vi "Lab Panel V4.82.vi"() -> ()   [LabVIEW 2013] (continued)
                        n2459 = call "sub vi - send mail with attach v5.vi"("TO:"=w4136, "subject"="MAIL TEST FROM LAB PANEL", "from"=w4135, "out going server"=w4134, "message"="TEST MESSAGE") -> ("error out"=w4138:errorcluster)  [unwired: 10 in]
                      }
                      frame #3 {
                        n2460 = Bundle(cluster=w4143, "TEST MAIL"=FALSE, "TEST MAIL STATUS"="TEST END", "mail error"=w4139) -> (w4141:T7)  [unwired: 4 in]
                        n2461 = local write "MAIL SETTINGS"(w4141) -> ()
                      }
                    }
                  }
                }
              }
              frame #1 {
                # "mail report"
                n2462 = stacked-sequence {
                  seq-local: [_ w4223 _ _] -> [_ _ _ w4391]
                  seq-local: [_ _ w4304 _] -> [_ _ _ w4381]
                  seq-local: [w4168 _ _ _] -> [_ w4217 _ _]
                  seq-local: [w4167 _ _ _] -> [_ w4216 _ _]
                  seq-local: [w4165 _ _ _] -> [_ w4214 _ _]
                  seq-local: [w4166 _ _ _] -> [_ w4215 _ _]
                  seq-local: [w4164 _ _ _] -> [_ w4213 _ _]
                  seq-local: [w4163 _ _ _] -> [_ w4208 _ _]
                  seq-local: [w4162 _ _ _] -> [_ w4209 _ _]
                  seq-local: [w4161 _ _ _] -> [_ w4210 _ _]
                  seq-local: [w4160 _ _ _] -> [_ w4211 _ _]
                  seq-local: [w4159 _ _ _] -> [_ w4212 _ _]
                  tunnel: w4158 -> [_ _ _ w4392]
                  tunnel: w4157 -> [_ _ _ w4375]
                  tunnel: w4156 -> [_ _ _ w4389]
                  tunnel: w4155 -> [_ _ _ w4388]
                  tunnel: w4154 -> [w4199 _ _ w4383]
                  tunnel: w4153 -> [_ _ w4334 _]
                  tunnel: w4152 -> [_ _ w4331 _]
                  tunnel: w4151 -> [_ _ w4330 _]
                  tunnel: w4150 -> [_ _ w4329 _]
                  tunnel: w4149 -> [_ _ w4328 _]
                  tunnel: w4148 -> [_ _ w4327 _]
                  tunnel: w4147 -> [_ _ w4326 _]
                  tunnel: w4146 -> [_ _ w4325 _]
                  tunnel: w4145 -> [_ _ w4324 _]
                  tunnel: w4144 -> [_ _ w4323 _]
                  frame #0 {
                    n2463 = case shown="False" w4199 {
                      frame False {
                        n2464 = local write "mail control"("") -> ()
                      }
                      frame True {
                      }
                    }
                    n2465 = local read "SET LAB01-1"() -> (w4198:T5)
                    n2466 = local read "SET LAB01-2"() -> (w4197:T5)
                    n2467 = local read "SET LAB02-1"() -> (w4196:T5)
                    n2468 = local read "SET LAB02-2"() -> (w4195:T5)
                    n2469 = local read "SET LAB03-1"() -> (w4194:T5)
                    n2470 = local read "SET LAB04-1"() -> (w4192:T5)
                    n2471 = local read "SET LAB05-1"() -> (w4190:T5)
                    n2472 = local read "SET LAB03-2"() -> (w4193:T5)
                    n2473 = local read "SET LAB04-2"() -> (w4191:T5)
                    n2474 = local read "SET LAB05-2"() -> (w4189:T5)
                    n2475 = Unbundle(w4194) -> ("DESCRIPTION"=w4174:string)  [unwired: 4 out]
                    n2476 = Unbundle(w4193) -> ("DESCRIPTION"=w4173:string)  [unwired: 4 out]
                    n2477 = Unbundle(w4192) -> ("DESCRIPTION"=w4172:string)  [unwired: 4 out]
                    n2478 = Unbundle(w4189) -> ("DESCRIPTION"=w4169:string)  [unwired: 4 out]
                    n2479 = Unbundle(w4195) -> ("DESCRIPTION"=w4175:string)  [unwired: 4 out]
                    n2480 = Unbundle(w4191) -> ("DESCRIPTION"=w4171:string)  [unwired: 4 out]
                    n2481 = Unbundle(w4198) -> ("DESCRIPTION"=w4187:string)  [unwired: 4 out]
                    n2482 = Unbundle(w4196) -> ("DESCRIPTION"=w4176:string)  [unwired: 4 out]
                    n2483 = Unbundle(w4190) -> ("DESCRIPTION"=w4170:string)  [unwired: 4 out]
                    n2484 = Unbundle(w4197) -> ("DESCRIPTION"=w4177:string)  [unwired: 4 out]
                    n2485 = Concatenate Strings("[LAB05-2/", w4169) -> (w4159:string)
                    n2486 = Concatenate Strings("[LAB05-1/", w4170) -> (w4160:string)
                    n2487 = Concatenate Strings("[LAB04-2/", w4171) -> (w4161:string)
                    n2488 = Concatenate Strings("[LAB03-2/", w4173) -> (w4163:string)
                    n2489 = Concatenate Strings("[LAB04-1/", w4172) -> (w4162:string)
                    n2490 = Concatenate Strings("[LAB03-1/", w4174) -> (w4164:string)
                    n2491 = Concatenate Strings("[LAB01-2/", w4177) -> (w4167:string)
                    n2492 = Concatenate Strings("[LAB02-2/", w4175) -> (w4165:string)
                    n2493 = Concatenate Strings("[LAB01-1/", w4187) -> (w4168:string)
                    n2494 = Concatenate Strings("[LAB02-1/", w4176) -> (w4166:string)
                  }
                  frame #1 {
                    w4221 = "/"
                    w4222 = 2.0
                    n2495 = local read "DISP LAB01-2"() -> (w4302:T4)
                    n2496 = local read "DISP LAB01-1"() -> (w4303:T4)
                    n2497 = local read "DISP LAB02-1"() -> (w4301:T4)
                    n2498 = local read "DISP LAB03-2"() -> (w4298:T4)
                    n2499 = local read "DISP LAB02-2"() -> (w4300:T4)
                    n2500 = local read "DISP LAB03-1"() -> (w4299:T4)
                    n2501 = local read "DISP LAB04-2"() -> (w4296:T4)
                    n2502 = local read "DISP LAB04-1"() -> (w4297:T4)
                    n2503 = local read "DISP LAB05-1"() -> (w4295:T4)
                    n2504 = local read "DISP LAB05-2"() -> (w4294:T4)
                    n2505 = Unbundle(w4302) -> ("CYCLE"=w4286:dbl, "MINS"=w4285:dbl, "STATUS"=w4282:string)
                    n2506 = Unbundle(w4303) -> ("CYCLE"=w4291:dbl, "MINS"=w4290:dbl, "STATUS"=w4287:string)
                    n2507 = Unbundle(w4301) -> ("CYCLE"=w4279:dbl, "MINS"=w4278:dbl, "STATUS"=w4277:string)
                    n2508 = Unbundle(w4298) -> ("CYCLE"=w4266:dbl, "MINS"=w4265:dbl, "STATUS"=w4262:string)
                    n2509 = Unbundle(w4299) -> ("CYCLE"=w4271:dbl, "MINS"=w4270:dbl, "STATUS"=w4267:string)
                    n2510 = Unbundle(w4300) -> ("CYCLE"=w4276:dbl, "MINS"=w4275:dbl, "STATUS"=w4272:string)
                    n2511 = Unbundle(w4297) -> ("CYCLE"=w4261:dbl, "MINS"=w4260:dbl, "STATUS"=w4257:string)
                    n2512 = Unbundle(w4296) -> ("CYCLE"=w4256:dbl, "MINS"=w4255:dbl, "STATUS"=w4252:string)
                    n2513 = Unbundle(w4295) -> ("CYCLE"=w4251:dbl, "MINS"=w4250:dbl, "STATUS"=w4247:string)
                    n2514 = Unbundle(w4294) -> ("CYCLE"=w4293:dbl, "MINS"=w4292:dbl, "STATUS"=w4244:string)
                    n2515 = Number To Decimal String(number=w4279) -> (decimal integer string=w4281:string)  [unwired: 1 in]
                    n2516 = Number To Decimal String(number=w4276) -> (decimal integer string=w4274:string)  [unwired: 1 in]
                    n2517 = Number To Decimal String(number=w4271) -> (decimal integer string=w4269:string)  [unwired: 1 in]
                    n2518 = Number To Decimal String(number=w4286) -> (decimal integer string=w4284:string)  [unwired: 1 in]
                    n2519 = Number To Decimal String(number=w4266) -> (decimal integer string=w4264:string)  [unwired: 1 in]
                    n2520 = Number To Decimal String(number=w4291) -> (decimal integer string=w4289:string)  [unwired: 1 in]
                    n2521 = Number To Decimal String(number=w4293) -> (decimal integer string=w4246:string)  [unwired: 1 in]
                    n2522 = Number To Decimal String(number=w4261) -> (decimal integer string=w4259:string)  [unwired: 1 in]
                    n2523 = Number To Decimal String(number=w4256) -> (decimal integer string=w4254:string)  [unwired: 1 in]
                    n2524 = Number To Decimal String(number=w4251) -> (decimal integer string=w4249:string)  [unwired: 1 in]
                    n2525 = Number To Fractional String(number=w4278, precision (6)=w4222) -> (F-format string=w4280:string)  [unwired: 2 in]
                    n2526 = Number To Fractional String(number=w4265, precision (6)=w4222) -> (F-format string=w4263:string)  [unwired: 2 in]
                    n2527 = Number To Fractional String(number=w4275, precision (6)=w4222) -> (F-format string=w4273:string)  [unwired: 2 in]
                    n2528 = Number To Fractional String(number=w4270, precision (6)=w4222) -> (F-format string=w4268:string)  [unwired: 2 in]
                    n2529 = Number To Fractional String(number=w4255, precision (6)=w4222) -> (F-format string=w4253:string)  [unwired: 2 in]
                    n2530 = Number To Fractional String(number=w4260, precision (6)=w4222) -> (F-format string=w4258:string)  [unwired: 2 in]
                    n2531 = Number To Fractional String(number=w4285, precision (6)=w4222) -> (F-format string=w4283:string)  [unwired: 2 in]
                    n2532 = Number To Fractional String(number=w4250, precision (6)=w4222) -> (F-format string=w4248:string)  [unwired: 2 in]
                    n2533 = Number To Fractional String(number=w4290, precision (6)=w4222) -> (F-format string=w4288:string)  [unwired: 2 in]
                    n2534 = Number To Fractional String(number=w4292, precision (6)=w4222) -> (F-format string=w4245:string)  [unwired: 2 in]
                    n2535 = Concatenate Strings(w4221, w4264, w4221, w4263, w4221, w4262) -> (w4238:string)
                    n2536 = Concatenate Strings(w4221, w4259, w4221, w4258, w4221, w4257) -> (w4237:string)
                    n2537 = Concatenate Strings(w4221, w4254, w4221, w4253, w4221, w4252) -> (w4236:string)
                    n2538 = Concatenate Strings(w4221, w4249, w4221, w4248, w4221, w4247) -> (w4235:string)
                    n2539 = Concatenate Strings(w4221, w4246, w4221, w4245, w4221, w4244) -> (w4234:string)
                    n2540 = Concatenate Strings(w4221, w4289, w4221, w4288, w4221, w4287) -> (w4243:string)
                    n2541 = Concatenate Strings(w4221, w4269, w4221, w4268, w4221, w4267) -> (w4239:string)
                    n2542 = Concatenate Strings(w4221, w4284, w4221, w4283, w4221, w4282) -> (w4242:string)
                    n2543 = Concatenate Strings(w4221, w4281, w4221, w4280, w4221, w4277) -> (w4241:string)
                    n2544 = Concatenate Strings(w4221, w4274, w4221, w4273, w4221, w4272) -> (w4240:string)
                    n2545 = Concatenate Strings("]", "\r") -> (w4218:string)
                    n2546 = Concatenate Strings(w4213, w4239, w4218) -> (w4229:string)
                    n2547 = Concatenate Strings(w4215, w4241, w4218) -> (w4231:string)
                    n2548 = Concatenate Strings(w4214, w4240, w4218) -> (w4230:string)
                    n2549 = Concatenate Strings(w4210, w4236, w4218) -> (w4226:string)
                    n2550 = Concatenate Strings(w4211, w4235, w4218) -> (w4227:string)
                    n2551 = Concatenate Strings(w4209, w4237, w4218) -> (w4225:string)
                    n2552 = Concatenate Strings(w4208, w4238, w4218) -> (w4224:string)
                    n2553 = Concatenate Strings(w4212, w4234, w4218) -> (w4228:string)
                    n2554 = Concatenate Strings(w4216, w4242, w4218) -> (w4232:string)
                    n2555 = Concatenate Strings(w4217, w4243, w4218) -> (w4233:string)
                    n2556 = Concatenate Strings(w4233, w4232, w4231, w4230, w4229, w4224, w4225, w4226, w4227, w4228) -> (w4201:string)
                    n2557 = Concatenate Strings("[PANEL/", "DESC/", "CYCLES/", "MINS/", "STATUS]", "\r", w4201) -> (w4223:string)
                    "MAIL REPORT" <- w4223
                  }
                  frame #2 {
                    w4332 = "END"
                    n2558 = local read "mail control"() -> (w4333:string)
                    n2559 = case shown="False" w4328 {
                      tunnel: w4333 -> [w4357 _]
                      tunnel: w4332 -> [w4356 _]
                      tunnel: [w4355 FALSE] -> w4318
                      frame False {
                        n2560 = Equal?(x=w4357, y=w4356) -> (x = y?=w4355:bool)
                      }
                      frame True {
                      }
                    }
                    n2561 = case shown="False" w4334 {
                      tunnel: w4333 -> [w4373 _]
                      tunnel: w4332 -> [w4372 _]
                      tunnel: [w4371 FALSE] -> w4322
                      frame False {
                        n2562 = Equal?(x=w4373, y=w4372) -> (x = y?=w4371:bool)
                      }
                      frame True {
                      }
                    }
                    n2563 = case shown="False" w4331 {
                      tunnel: w4333 -> [w4369 _]
                      tunnel: w4332 -> [w4368 _]
                      tunnel: [w4367 FALSE] -> w4321
                      frame False {
                        n2564 = Equal?(x=w4369, y=w4368) -> (x = y?=w4367:bool)
                      }
                      frame True {
                      }
                    }
                    n2565 = case shown="False" w4329 {
                      tunnel: w4333 -> [w4361 _]
                      tunnel: w4332 -> [w4360 _]
                      tunnel: [w4359 FALSE] -> w4319
                      frame False {
                        n2566 = Equal?(x=w4361, y=w4360) -> (x = y?=w4359:bool)
                      }
                      frame True {
                      }
                    }
                    n2567 = case shown="False" w4330 {
                      tunnel: w4333 -> [w4365 _]
                      tunnel: w4332 -> [w4364 _]
                      tunnel: [w4363 FALSE] -> w4320
                      frame False {
                        n2568 = Equal?(x=w4365, y=w4364) -> (x = y?=w4363:bool)
                      }
                      frame True {
                      }
                    }
                    n2569 = Or(x=w4320, y=w4319) -> (x .or. y?=w4311:bool)
                    n2570 = Or(x=w4322, y=w4321) -> (x .or. y?=w4312:bool)
                    n2571 = Or(x=w4312, y=w4311) -> (x .or. y?=w4307:bool)
                    n2572 = case shown="False" w4324 {
                      tunnel: w4333 -> [w4341 _]
                      tunnel: w4332 -> [w4340 _]
                      tunnel: [w4339 FALSE] -> w4313
                      frame False {
                        n2573 = Equal?(x=w4341, y=w4340) -> (x = y?=w4339:bool)
                      }
                      frame True {
                      }
                    }
                    n2574 = case shown="False" w4323 {
                      tunnel: w4333 -> [w4337 _]
                      tunnel: w4332 -> [w4336 _]
                      tunnel: [w4335 FALSE] -> w4317
                      frame False {
                        n2575 = Equal?(x=w4337, y=w4336) -> (x = y?=w4335:bool)
                      }
                      frame True {
                      }
                    }
                    n2576 = case shown="False" w4325 {
                      tunnel: w4333 -> [w4345 _]
                      tunnel: w4332 -> [w4344 _]
                      tunnel: [w4343 FALSE] -> w4314
                      frame False {
                        n2577 = Equal?(x=w4345, y=w4344) -> (x = y?=w4343:bool)
                      }
                      frame True {
                      }
                    }
                    n2578 = case shown="False" w4327 {
                      tunnel: w4333 -> [w4353 _]
                      tunnel: w4332 -> [w4352 _]
                      tunnel: [w4351 FALSE] -> w4316
                      frame False {
                        n2579 = Equal?(x=w4353, y=w4352) -> (x = y?=w4351:bool)
                      }
                      frame True {
                      }
                    }
                    n2580 = case shown="False" w4326 {
                      tunnel: w4333 -> [w4349 _]
                      tunnel: w4332 -> [w4348 _]
                      tunnel: [w4347 FALSE] -> w4315
                      frame False {
                        n2581 = Equal?(x=w4349, y=w4348) -> (x = y?=w4347:bool)
                      }
                      frame True {
                      }
                    }
                    n2582 = Or(x=w4316, y=w4315) -> (x .or. y?=w4310:bool)
                    n2583 = Or(x=w4314, y=w4313) -> (x .or. y?=w4309:bool)
                    n2584 = Or(x=w4317, y=w4318) -> (x .or. y?=w4305:bool)
                    n2585 = Or(x=w4310, y=w4309) -> (x .or. y?=w4308:bool)
                    n2586 = Or(x=w4307, y=w4308) -> (x .or. y?=w4306:bool)
                    n2587 = Or(x=w4306, y=w4305) -> (x .or. y?=w4304:bool)
                  }
                  frame #3 {
                    n2588 = local read "on loops"() -> (w4387:dbl)
                    n2589 = local read "jig cycle"() -> (w4384:dbl)
                    n2590 = local read "Send Mail Now"() -> (w4378:bool)
                    n2591 = Add(x=w4387, y=3.0) -> (x+y=w4385:dbl)
                    n2592 = Equal?(x=w4384, y=w4385) -> (x = y?=w4379:bool)
                    n2593 = And(x=w4379, y=w4378) -> (x .and. y?=w4377:bool)
                    n2594 = And(x=w4383, y=w4379) -> (x .and. y?=w4382:bool)
                    n2595 = And(x=w4382, y=w4381) -> (x .and. y?=w4380:bool)
                    n2596 = Or(x=w4380, y=w4377) -> (x .or. y?=w4376:bool)
                    n2597 = case shown="True" w4376 {
                      tunnel: w4392 -> [_ w4398]
                      tunnel: w4391 -> [_ w4397]
                      tunnel: "Lab Panel Test Status" -> [_ w4396]
                      tunnel: w4389 -> [_ w4395]
                      tunnel: w4388 -> [_ w4394]
                      tunnel: w4375 -> [_ w4393]
                      frame False {
                      }
                      frame True {
                        n2598 = stacked-sequence {
                          tunnel: w4398 -> [w4406 _]
                          tunnel: w4397 -> [w4405 _]
                          tunnel: w4396 -> [w4404 _]
                          tunnel: w4395 -> [w4403 _]
                          tunnel: w4394 -> [w4402 _]
                          tunnel: w4393 -> [w4401 _]
                          frame #0 {
                            n2599 = call "sub vi - send mail with attach v5.vi"("TO:"=w4406, "subject"=w4404, "from"=w4402, "out going server"=w4403, "message"=w4405) -> ("error out"=w4400:errorcluster)  [unwired: 10 in]
                            n2600 = Bundle(cluster=w4401, "mail error"=w4400) -> (w4399:T7)  [unwired: 6 in]
                            n2601 = local write "MAIL SETTINGS"(w4399) -> ()
                          }
                          frame #1 {
                            n2602 = local write "mail control"("") -> ()
                            n2603 = local write "Send Mail Now"(FALSE) -> ()
                          }
                        }
                      }
                    }
                  }
                }
              }
            }
          }
          frame #18 {
            # "save jig cycle values once all run switches are off"
            n2604 = stacked-sequence {
              tunnel: w4418 -> [_ w4447]
              tunnel: w4417 -> [_ w4446]
              tunnel: w4416 -> [_ w4445]
              tunnel: w4415 -> [_ w4444]
              tunnel: w4414 -> [_ w4443]
              tunnel: w4413 -> [_ w4442]
              tunnel: w4412 -> [_ w4441]
              tunnel: w4411 -> [_ w4440]
              tunnel: w4410 -> [_ w4439]
              tunnel: w4409 -> [_ w4438]
              frame #0 {
              }
              frame #1 {
                n2605 = Not(x=w4438) -> (.not. x?=w4421:bool)
                n2606 = Not(x=w4446) -> (.not. x?=w4436:bool)
                n2607 = Not(x=w4443) -> (.not. x?=w4431:bool)
                n2608 = Not(x=w4441) -> (.not. x?=w4427:bool)
                n2609 = Not(x=w4439) -> (.not. x?=w4423:bool)
                n2610 = Not(x=w4447) -> (.not. x?=w4437:bool)
                n2611 = Not(x=w4445) -> (.not. x?=w4435:bool)
                n2612 = Not(x=w4442) -> (.not. x?=w4429:bool)
                n2613 = Not(x=w4444) -> (.not. x?=w4433:bool)
                n2614 = Not(x=w4440) -> (.not. x?=w4425:bool)
                n2615 = local read "Save JC"() -> (w4449:bool)
                n2616 = And(x=w4437, y=w4436) -> (x .and. y?=w4434:bool)
                n2617 = And(x=w4434, y=w4435) -> (x .and. y?=w4432:bool)
                n2618 = And(x=w4432, y=w4433) -> (x .and. y?=w4430:bool)
                n2619 = And(x=w4430, y=w4431) -> (x .and. y?=w4428:bool)
                n2620 = And(x=w4428, y=w4429) -> (x .and. y?=w4426:bool)
                n2621 = And(x=w4426, y=w4427) -> (x .and. y?=w4424:bool)
                n2622 = And(x=w4424, y=w4425) -> (x .and. y?=w4422:bool)
                n2623 = And(x=w4422, y=w4423) -> (x .and. y?=w4420:bool)
                n2624 = And(x=w4420, y=w4421) -> (x .and. y?=w4419:bool)
                n2625 = And(x=w4419, y=w4449) -> (x .and. y?=w4448:bool)
                n2626 = case shown="True" w4448 {
                  tunnel: w4419 -> [w4450 _]
                  frame False {
                    n2627 = case shown="False" w4450 {
                      frame False {
                        n2628 = local write "Save JC"(TRUE) -> ()
                      }
                      frame True {
                      }
                    }
                  }
                  frame True {
                    n2629 = stacked-sequence {
                      frame #0 {
                        n2630 = String To Path(string="c:\\crabtree\\Jig Cycles\\") -> (path=w4462:path)
                        n2631 = Build Path(base path=w4462, name or relative path="jigcycles.bin") -> (appended path=w4460:path)
                        n2632 = Create Folder(path (use dialog)=w4462) -> (error out=w4464:errorcluster)  [unwired: 2 in, 2 out]
                        n2633 = local read "JIG RELAY CYCLES"() -> (w4454:T10)
                        n2634 = call <vilib>:"Clear Errors.vi"("error in (no error)"=w4464) -> ()  [unwired: 6 in, 1 out]
                        n2635 = local write "Save JC"(FALSE) -> ()
                        n2636 = Open/Create/Replace File(file path (use dialog)=w4460, operation (0:open)=T20."replace or create") -> (refnum out=w4458:refnum<file>, error out=w4459:errorcluster)  [unwired: 4 in, 1 out]
                        n2637 = Write to Binary File(file (use dialog)=w4458, data=w4454, error in=w4459) -> (refnum out=w4457:refnum<file>, error out=w4456:errorcluster)  [unwired: 3 in, 1 out]
                        n2638 = Close File(refnum=w4457, error in=w4456) -> (error out=w4455:errorcluster)  [unwired: 1 out]
                        n2639 = local write "data file error"(w4455) -> ()
                      }
                      frame #1 {
                        n2640 = local read "JIG RELAY CYCLES"() -> (w4487:T10)
                        n2641 = Unbundle By Name(w4487) -> ("LAB01-1"=w4482:dbl, "LAB01-2"=w4481:dbl, "LAB02-1"=w4479:dbl, "LAB02-2"=w4478:dbl, "LAB03-1"=w4476:dbl, "LAB03-2"=w4473:dbl, "LAB04-1"=w4472:dbl, "LAB04-2"=w4470:dbl, "LAB05-1"=w4468:dbl, "LAB05-2"=w4466:dbl)
                        n2642 = stacked-sequence {
                          tunnel: w4482 -> [w4490 _ _ _ _ _ _ _ _ _]
                          tunnel: 1000000 -> [w4493 w4503 w4513 w4523 w4533 w4543 w4553 w4563 w4573 w4583]
                          tunnel: [w4491 _ _ _ _ _ _ _ _ _] -> w4485
                          tunnel: "TEST STATION HAS REACHED 1 MILLION CYCLES, REPLACE  CONTROL RELAYS" -> [w4489 w4501 w4511 w4521 w4531 w4541 w4551 w4561 w4571 w4581]
                          tunnel: [_ w4500 _ _ _ _ _ _ _ _] -> w4483
                          tunnel: w4481 -> [_ w4499 _ _ _ _ _ _ _ _]
                          tunnel: [_ _ w4510 _ _ _ _ _ _ _] -> w4480
                          tunnel: w4479 -> [_ _ w4509 _ _ _ _ _ _ _]
                          tunnel: w4478 -> [_ _ _ w4520 _ _ _ _ _ _]
                          tunnel: [_ _ _ w4519 _ _ _ _ _ _] -> w4477
                          tunnel: w4476 -> [_ _ _ _ w4530 _ _ _ _ _]
                          tunnel: [_ _ _ _ w4529 _ _ _ _ _] -> w4475
                          tunnel: [_ _ _ _ _ w4540 _ _ _ _] -> w4474
                          tunnel: w4473 -> [_ _ _ _ _ w4539 _ _ _ _]
                          tunnel: w4472 -> [_ _ _ _ _ _ w4550 _ _ _]
                          tunnel: [_ _ _ _ _ _ w4549 _ _ _] -> w4471
                          tunnel: w4470 -> [_ _ _ _ _ _ _ w4560 _ _]
                          tunnel: [_ _ _ _ _ _ _ w4559 _ _] -> w4469
                          tunnel: w4468 -> [_ _ _ _ _ _ _ _ w4570 _]
                          tunnel: [_ _ _ _ _ _ _ _ w4569 _] -> w4467
                          tunnel: w4466 -> [_ _ _ _ _ _ _ _ _ w4580]
                          tunnel: [_ _ _ _ _ _ _ _ _ w4579] -> w4465
                          frame #0 {
